vi "Init Lockin.vi"(8 "error in (no error)":errorcluster, 11 "DAQmx Lockin Digitizer Driver in":refnum<class "DAQmx Lockin Digitizer Driver.lvclass">) -> (0 "error out":errorcluster, 3 "DAQmx Lockin Digitizer Driver out":refnum<class "DAQmx Lockin Digitizer Driver.lvclass">)   [LabVIEW 2021, in "DAQmx Lockin Digitizer Driver.lvclass"]
uses:
  DAQmx Lockin Digitizer Driver.lvclass
  C:/GitHub/NHMFL_Core/Libraries/NI-DAQ/DAQmx Digitizer/DAQmx Digitizer.lvclass
  DAQmx Lockin Digitizer Driver.lvclass/DAQmx Lockin Digitizer Driver.ctl
  <resource>/objmgr/daqmx.rc
panel:
  out "ChannelsToRead":refnum<k21>
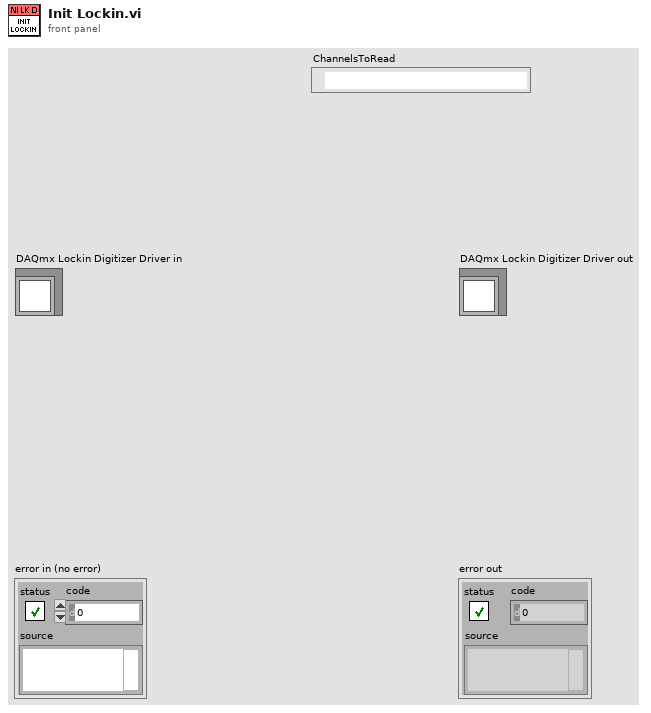
[diagram p1: front panel]
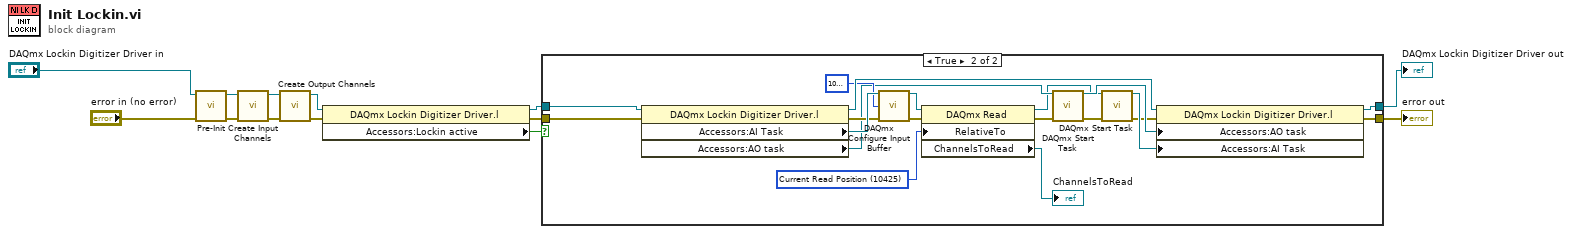
[diagram p0: block diagram]
diagram:
  n1 = call-dynamic "Pre-Init.vi"("error in (no error)"="error in (no error)", "DAQmx Lockin Digitizer Driver in"="DAQmx Lockin Digitizer Driver in") -> ("error out"=w13:errorcluster, "DAQmx Lockin Digitizer Driver out"=w10:refnum<class "DAQmx Lockin Digitizer Driver.lvclass">)  [unwired: 8 in]
  n2 = call-dynamic "Create Input Channels.vi"("error in (no error)"=w13, "DAQmx Digitizer in"=w10) -> ("error out"=w8:errorcluster, "DAQmx Digitizer out"=w9:refnum<class "DAQmx Lockin Digitizer Driver.lvclass">)  [unwired: 8 in]
  n3 = call-dynamic "Create Output Channels.vi"("error in (no error)"=w8, "DAQmx Lockin Digitizer Driver in"=w9) -> ("error out"=w5:errorcluster, "DAQmx Lockin Digitizer Driver out"=w2:refnum<class "DAQmx Lockin Digitizer Driver.lvclass">)  [unwired: 8 in]
  n4 = property class="DAQmx Lockin Digitizer Driver.l"(reference=w2, error in=w5) -> (reference out=w3:refnum<class "DAQmx Lockin Digitizer Driver.lvclass">, error out=w1:errorcluster, "Accessors:Lockin active"=w4:bool)
  n5 = case shown="True" w4 {
    tunnel: w1 -> [w14 w27]
    tunnel: [w15 w19] -> w7
    tunnel: [w14 w18] -> w6
    tunnel: w3 -> [w15 w17]
    frame False {
    }
    frame True {
      w29 = 10425 items=["First Sample"=10424, "Current Read Position"=10425, "Reference Trigger"=10426, "First Pretrigger Sample"=10427, "Most Recent Sample"=10428] ("RelativeTo")
      n6 = property class="DAQmx Lockin Digitizer Driver.l"(reference=w17, error in=w27) -> (reference out=w34:refnum<class "DAQmx Lockin Digitizer Driver.lvclass">, error out=w31:errorcluster, "Accessors:AI Task"=w33:refnum<k21>, "Accessors:AO task"=w26:refnum<k21>)
      n7 = call <vilib>:"DAQmx Configure Input Buffer.vi"("task/channels in"=w33, "buffer size (in samples per channel)"=u32 1000000, "error in"=w31) -> ("task out"=w30:refnum<k21>, "error out"=w28:errorcluster)  [unwired: 11 in]
      n8 = property class="DAQmx Read"(reference=w30, error in=w28, "RelativeTo"=w29) -> (reference out=w23:refnum<k21>, error out=w25:errorcluster, "ChannelsToRead"=→"ChannelsToRead":refnum<k21>)
      n9 = call <vilib>:"DAQmx Start Task.vi"("task/channels in"=w26, "error in"=w25) -> ("task out"=w24:refnum<k21>, "error out"=w21:errorcluster)  [unwired: 12 in]
      n10 = call <vilib>:"DAQmx Start Task.vi"("task/channels in"=w23, "error in"=w21) -> ("task out"=w22:refnum<k21>, "error out"=w20:errorcluster)  [unwired: 12 in]
      n11 = property class="DAQmx Lockin Digitizer Driver.l"(reference=w34, error in=w20, "Accessors:AO task"=w24, "Accessors:AI Task"=w22) -> (reference out=w19:refnum<class "DAQmx Lockin Digitizer Driver.lvclass">, error out=w18:errorcluster)
    }
  }
  "error out" <- w6
  "DAQmx Lockin Digitizer Driver out" <- w7
